vi "UTILITY Array Reset.vi"(7 "Reset After 24hrs":bool=TRUE, 11 "Plot Array Input":dbl[][](array[numeric])) -> (3 "Reset Array":bool)   [LabVIEW 2020]
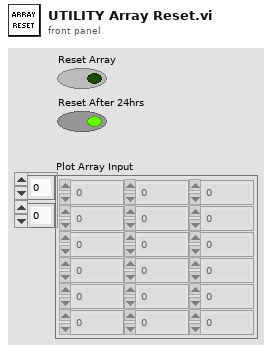
[diagram p1: front panel]
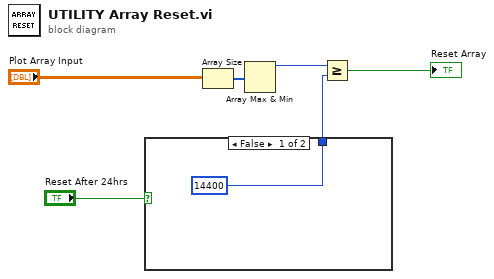
[diagram p0: block diagram]
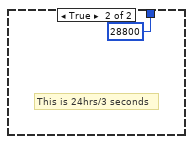
[diagram p2: hidden frame]
diagram:
  n1 = case shown="False" "Reset After 24hrs" {
    tunnel: [14400 ("y") 28800 ("y")] -> w5
    frame False {
    }
    frame True {
      # "This is 24hrs/3 seconds"
    }
  }
  n2 = Array Size(array="Plot Array Input") -> (size(s)=w3:i32[])
  n3 = Array Max & Min(array=w3) -> (max value=w4:i32)  [unwired: 3 out]
  n4 = Greater Or Equal?(x=w4, y=w5) -> (x >= y?=→"Reset Array":bool)
